vi "FTW-TransferClient-Cancel.vi"(0 "Transfer Client":refnum<class "FTW-TransferClient-S3.lvclass">, 11 "error in":errorcluster) -> (4 "Transfer Client out":refnum<class "FTW-TransferClient-S3.lvclass">, 15 "error out":errorcluster)   [LabVIEW 2014, in "FTW-TransferClient-S3.lvclass"]
uses:
  FTW-TransferClient-S3.lvclass
  C:/Users/Jack/repo/ftw-master/ftw/src/windows/transfer/S3/AWSSDK.dll
  AWSSDK.dll
  FTW-TransferClient.lvclass
panel:
  # "Inputs"
  # "Outputs"
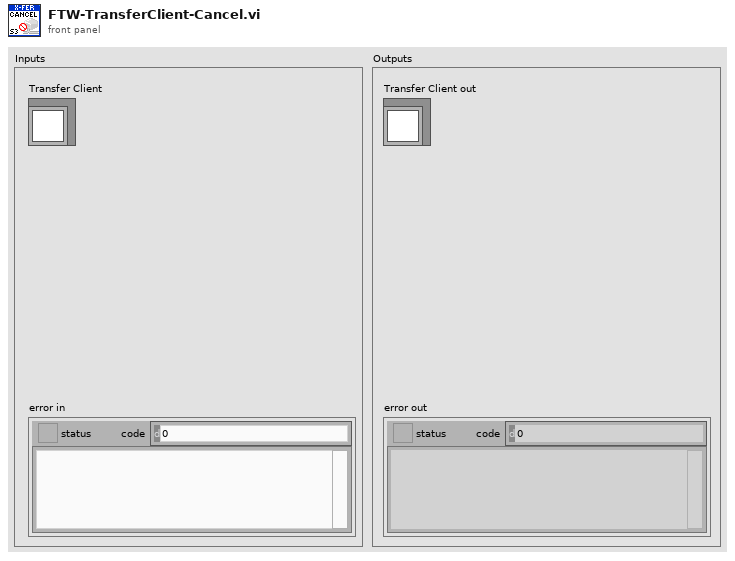
[diagram p1: front panel]
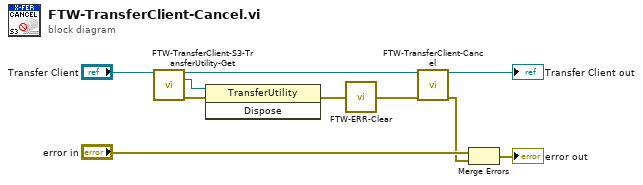
[diagram p0: block diagram]
diagram:
  n1 = call "FTW-TransferClient-S3-TransferUtility-Get.vi"("Transfer Client"="Transfer Client") -> ("Transfer Client out"=w5:refnum<class "FTW-TransferClient-S3.lvclass">, "Transfer Utility ref"=w4:refnum<k24>, "error out"=w3:errorcluster)  [unwired: 12 in]
  n2 = invoke class="TransferUtility" method="Dispose"(reference=w4, error in=w3) -> (error out=w2:errorcluster)  [unwired: 1 in, 2 out]
  n3 = call "FTW-ERR-Clear.vi"("error to snuff"=w2) -> ("no error"=w1:errorcluster)
  n4 = call-parent "FTW-TransferClient-Cancel.vi"("Transfer Client"=w5, "error in"=w1) -> ("Transfer Client out"=→"Transfer Client out":refnum<class "FTW-TransferClient-S3.lvclass">, "error out"=w8:errorcluster)  [unwired: 12 in]
  n5 = Merge Errors("error in", w8) -> (→"error out":errorcluster)
